vi "P2-3.vi"() -> ()   [LabVIEW 2011]
panel:
  out "불리언":bool
  out "X/Y":dbl
  out "X*Y":dbl
  in  "Y":dbl
  in  "X":dbl
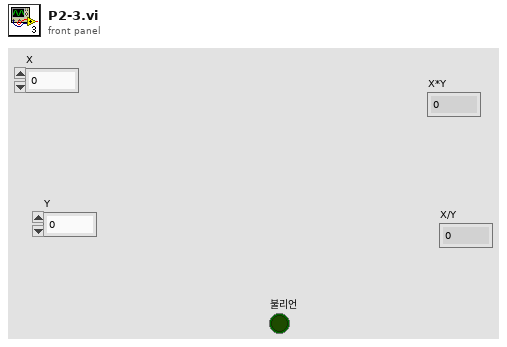
[diagram p1: front panel]
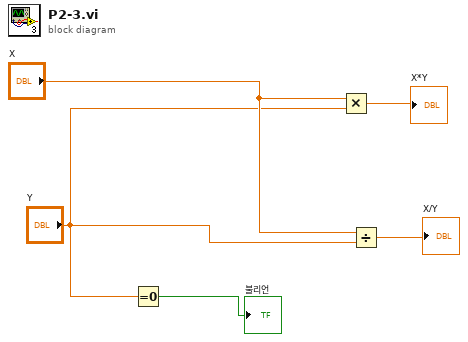
[diagram p0: block diagram]
diagram:
  n1 = Equal To 0?(x="Y") -> (x = 0?=→"불리언":bool)
  n2 = Multiply(x="X", y="Y") -> (x*y=→"X*Y":dbl)
  n3 = Divide(x="X", y="Y") -> (x/y=→"X/Y":dbl)
